vi "derivative_power.vi"(0 "Temp":dbl, 7 "Control Parameters":T1={"Setpoint"=50.0, "Control bandwidth"=4.0, "Settle bandwidth"=1.0, "Integral time"=30.0, "Int\non"=TRUE, "Derivative time"=0.5, "Der\non"=TRUE, "Settle time"=60.0} {"Settle time" format="%.2f"; "Derivative time" format="%.2f"; "Integral time" format="%.2f"; "Settle bandwidth" format="%.2f"; "Control bandwidth" format="%.2f"; "Setpoint" format="%.2f"}, 11 "Reset PID":bool, 13 "Elapsed Time":dbl) -> (4 "Normalized Power":dbl)   [LabVIEW 2016]
uses:
  typedefs/control parameters.ctl
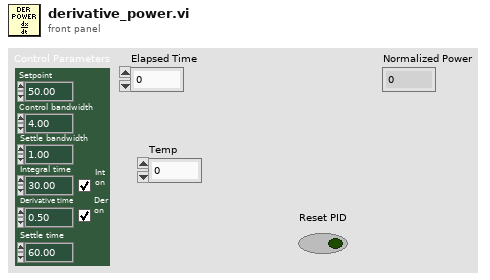
[diagram p1: front panel]
types:
  T1 = typedef "control parameters.ctl" = cluster{"Setpoint":dbl, "Control bandwidth":dbl, "Settle bandwidth":dbl, "Integral time":dbl, "Int\non":bool, "Derivative time":dbl, "Der\non":bool, "Settle time":dbl}
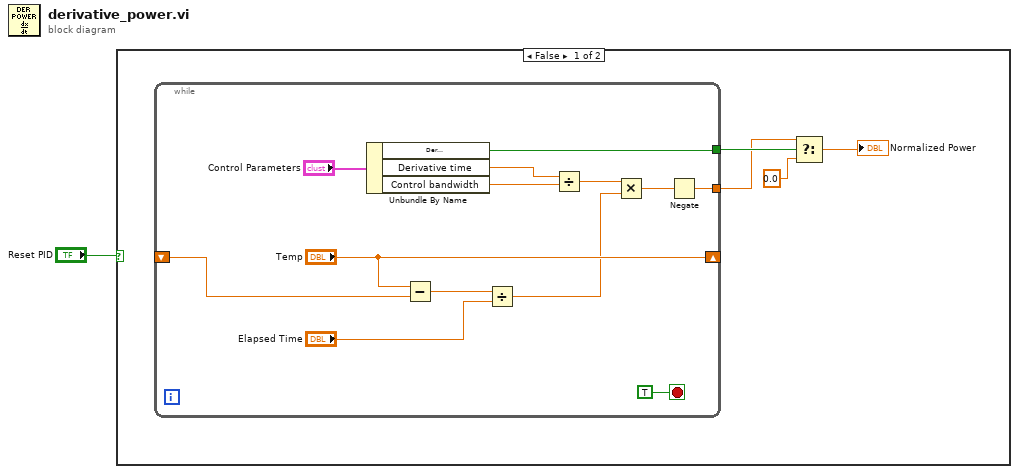
[diagram p0: block diagram]
diagram:
  n1 = case shown="False" "Reset PID" {
    frame False {
      n2 = while {
        shift-right: ["Temp"] -> _
        shift-left: _ -> [w15]
        tunnel: [w7] -> w4
        tunnel: [w6] -> w3
        stop <- TRUE stop-if-true
        n3 = Unbundle By Name("Control Parameters") -> ("Der\non"=w7:bool, "Derivative time"=w12:dbl, "Control bandwidth"=w13:dbl)
        n4 = Subtract(x="Temp", y=w15) -> (x-y=w14:dbl)
        n5 = Divide(x=w14, y="Elapsed Time") -> (x/y=w11:dbl)
        n6 = Divide(x=w12, y=w13) -> (x/y=w10:dbl)
        n7 = Multiply(x=w10, y=w11) -> (x*y=w9:dbl)
        n8 = Negate(x=w9) -> (-x=w6:dbl)
      }
      n9 = Select(t=w3, s=w4, f=0.0) -> (s? t:f=→"Normalized Power":dbl)
    }
    frame True {
    }
  }
